vi "16DUT VSA Plot Ver1.0.vi"(6 "Plot":T1(ring), 7 "No of Rows":i32=10496, 8 "error in (no error)":errorcluster, 10 "Bank":enum16{"C1", "C2", "C3"}(ring), 11 "file path (dialog if empty)":path) -> (0 "error out":errorcluster, 3 "Delta C_Min Plot":dbl[][](graph) caption="(Y) Multi Plot 2")   [LabVIEW 2012]
uses:
  <vilib>/Utility/file.llb/Read From Spreadsheet File (string).vi
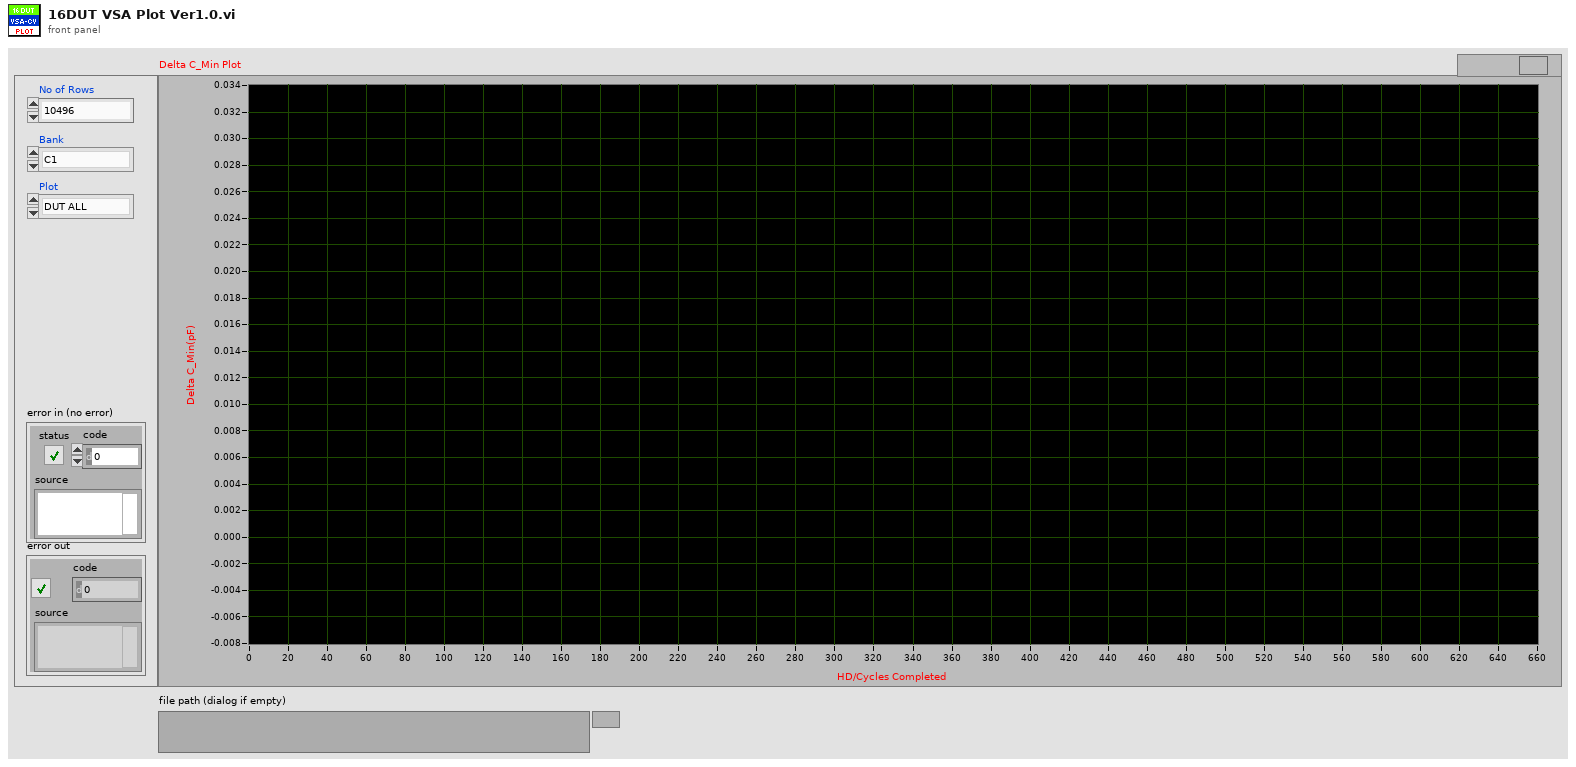
[diagram p1: front panel]
types:
  T1 = enum16{"DUT ALL", "DUT 01", "DUT 02", "DUT 03", "DUT 04", "DUT 05", "DUT 06", "DUT 07", "DUT 08", "DUT 09", "DUT 10", "DUT 11", "DUT 12", "DUT 13", "DUT 14", "DUT 15", "DUT 16"}
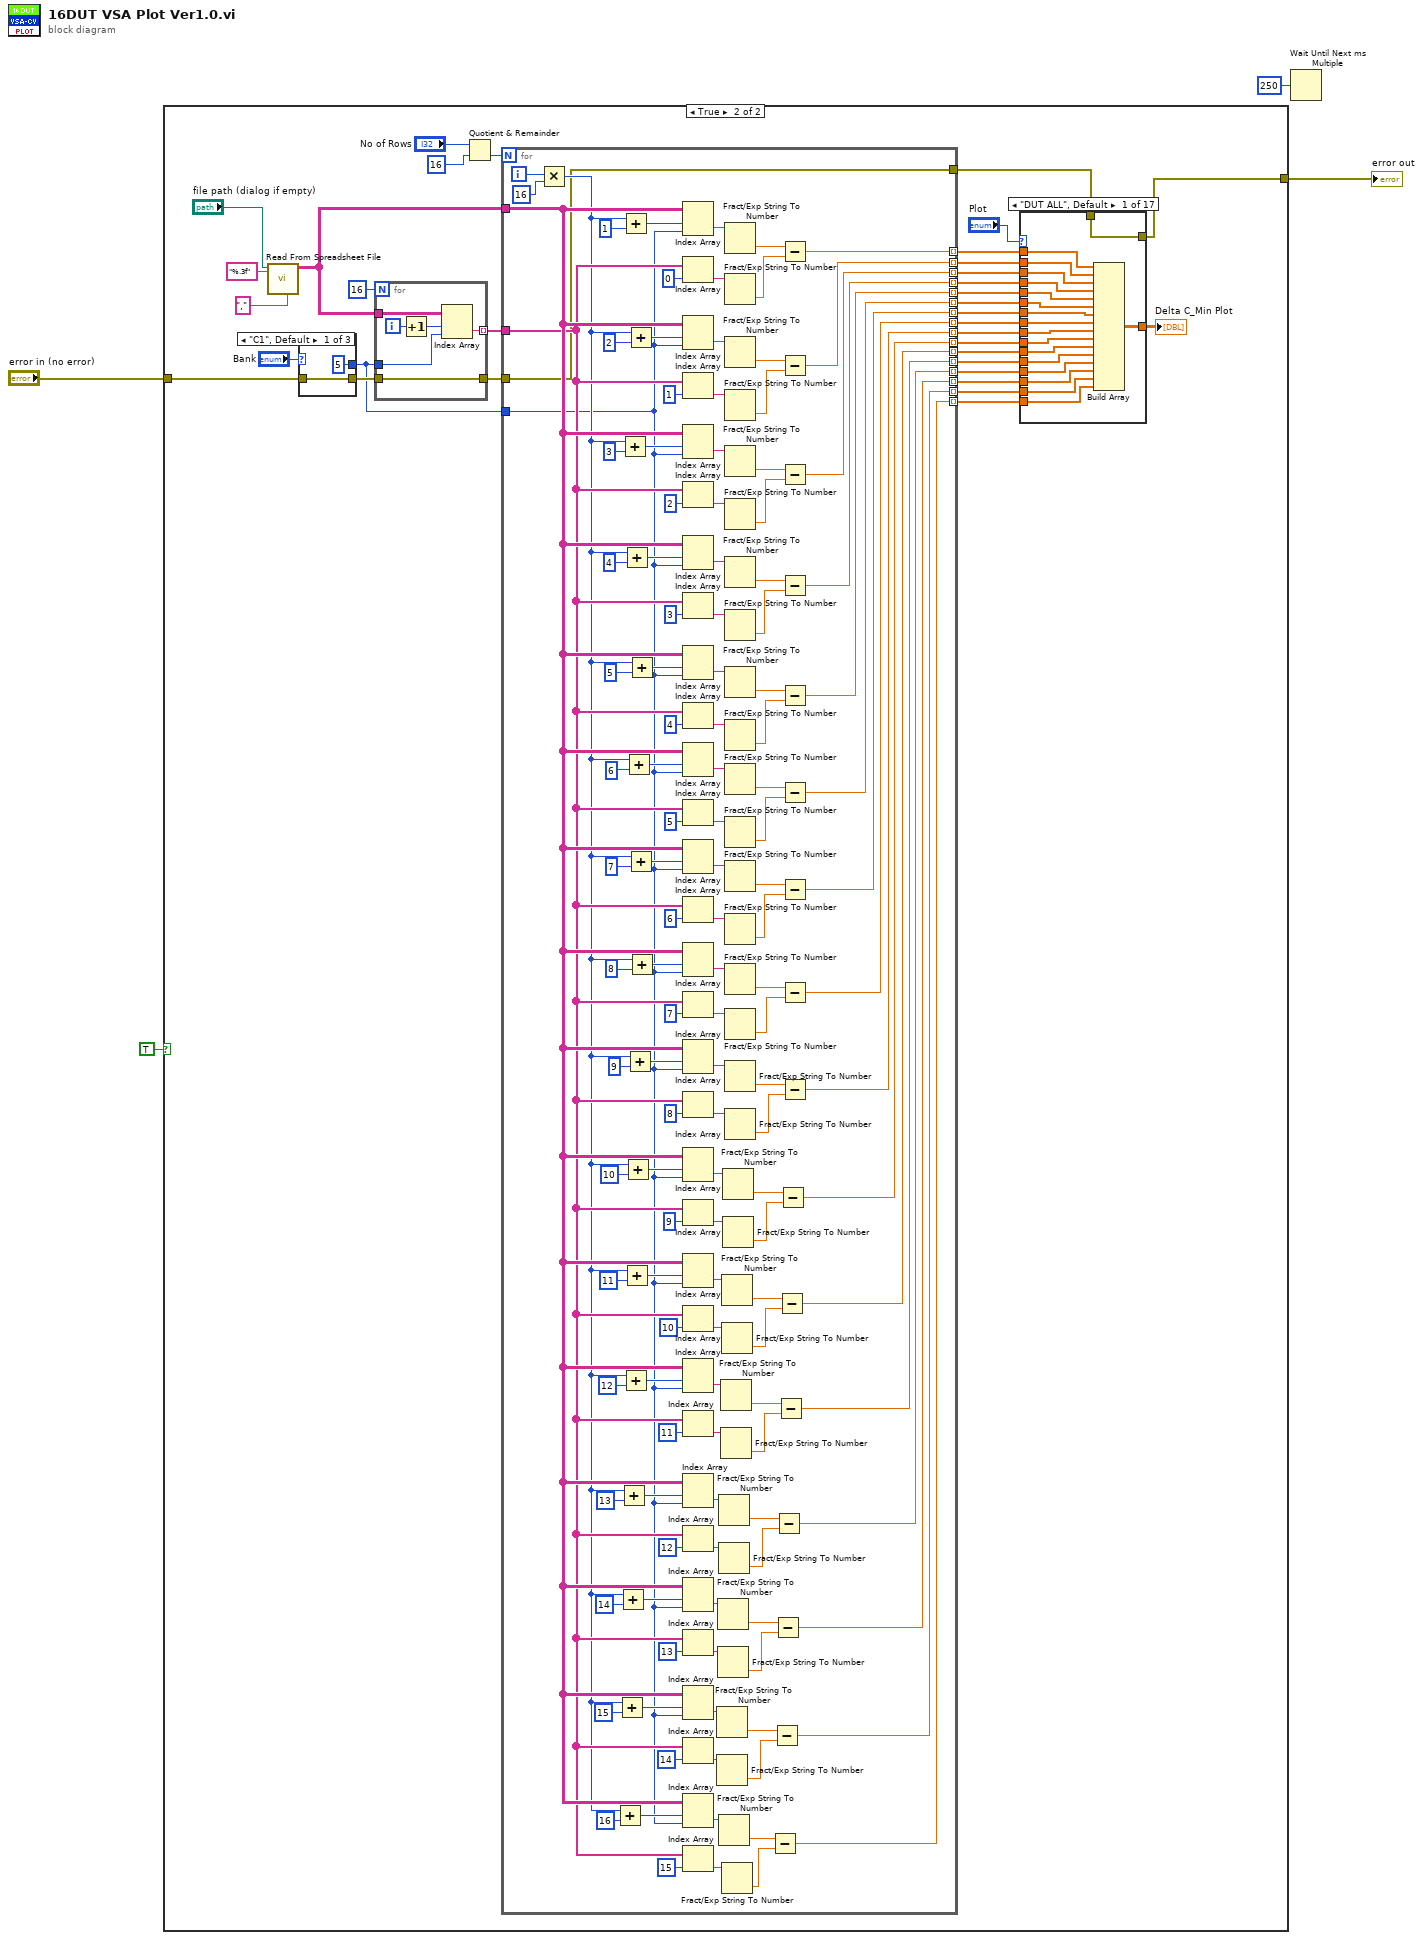
[diagram p0: block diagram]
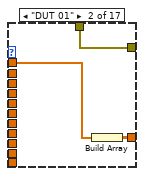
[diagram p3: hidden frame]
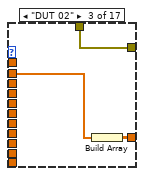
[diagram p4: hidden frame]
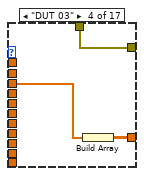
[diagram p5: hidden frame]
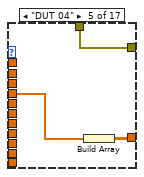
[diagram p6: hidden frame]
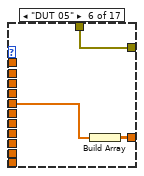
[diagram p7: hidden frame]
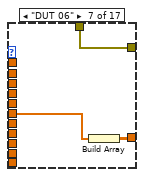
[diagram p8: hidden frame]
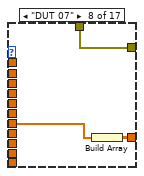
[diagram p9: hidden frame]
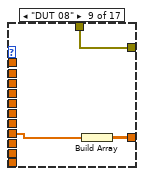
[diagram p10: hidden frame]
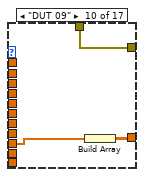
[diagram p11: hidden frame]
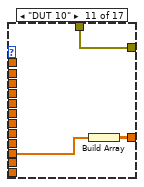
[diagram p12: hidden frame]
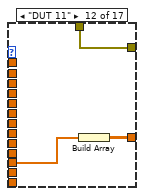
[diagram p13: hidden frame]
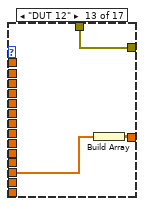
[diagram p14: hidden frame]
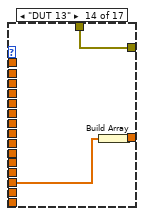
[diagram p15: hidden frame]
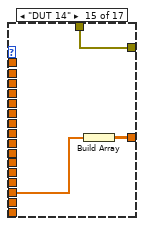
[diagram p16: hidden frame]
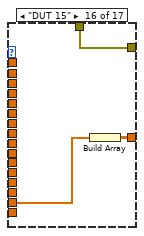
[diagram p17: hidden frame]
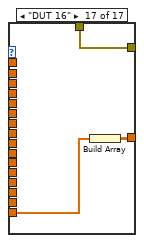
[diagram p18: hidden frame]
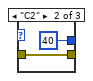
[diagram p19: hidden frame]
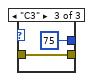
[diagram p20: hidden frame]
diagram:
  n1 = case shown="True" TRUE {
    tunnel: "error in (no error)" -> [w5 w12]
    tunnel: [w5 w6] -> w3
    frame False {
    }
    frame True {
      n2 = call-poly <vilib>:"Read From Spreadsheet File.vi"("delimiter (\\t)"="," ("delimiter (\\t)"), "format (%s)"="%.3f" ("format (%.3f)"), "file path (dialog if empty)"="file path (dialog if empty)") -> ("all rows"=w36:string[][])  [unwired: 4 in, 4 out]
      n3 = case shown="\"C1\", Default" "Bank" {
        tunnel: [5 40 75] -> w8
        tunnel: [w106 w108 w110] -> w9
        tunnel: w12 -> [w106 w108 w110]
        frame "C1", Default {
        }
        frame "C2" {
        }
        frame "C3" {
        }
      }
      n4 = for {
        N: 16 -> [_]
        tunnel: w36 -> [w252]
        tunnel: [w251] -> w35 mode=indexing
        tunnel: w8 -> [w247]
        tunnel: [w248] -> w11
        tunnel: w9 -> [w248]
        i -> [w250]
        n5 = Increment(x=w250) -> (x+1=w249:i32)
        n6 = Index Array(array=w252, index (row)=w249, index (col)=w247) -> (element=w251:string)
      }
      n7 = Quotient & Remainder(x="No of Rows", y=16) -> (floor(x/y)=w31:i32)  [unwired: 1 out]
      n8 = for {
        N: w31 -> [_]
        tunnel: w36 -> [w133]
        tunnel: w35 -> [w132]
        tunnel: [w130] -> w29 mode=indexing
        tunnel: [w129] -> w28 mode=indexing
        tunnel: [w128] -> w27 mode=indexing
        tunnel: [w127] -> w26 mode=indexing
        tunnel: [w126] -> w25 mode=indexing
        tunnel: [w125] -> w24 mode=indexing
        tunnel: [w124] -> w23 mode=indexing
        tunnel: [w123] -> w22 mode=indexing
        tunnel: [w122] -> w21 mode=indexing
        tunnel: [w121] -> w20 mode=indexing
        tunnel: [w120] -> w19 mode=indexing
        tunnel: [w119] -> w18 mode=indexing
        tunnel: [w118] -> w17 mode=indexing
        tunnel: [w117] -> w16 mode=indexing
        tunnel: [w116] -> w15 mode=indexing
        tunnel: [w115] -> w14 mode=indexing
        tunnel: w11 -> [w114]
        tunnel: [w114] -> w10
        tunnel: w8 -> [w113]
        i -> [w112]
        n9 = Multiply(x=w112, y=16) -> (x*y=w131:i32)
        n10 = Add(x=w131, y=16) -> (x+y=w138:i32)
        n11 = Add(x=w131, y=15) -> (x+y=w143:i32)
        n12 = Add(x=w131, y=14) -> (x+y=w152:i32)
        n13 = Add(x=w131, y=13) -> (x+y=w157:i32)
        n14 = Add(x=w131, y=3) -> (x+y=w212:i32)
        n15 = Add(x=w131, y=1) -> (x+y=w234:i32)
        n16 = Add(x=w131, y=12) -> (x+y=w166:i32)
        n17 = Add(x=w131, y=4) -> (x+y=w211:i32)
        n18 = Add(x=w131, y=11) -> (x+y=w171:i32)
        n19 = Add(x=w131, y=10) -> (x+y=w180:i32)
        n20 = Add(x=w131, y=6) -> (x+y=w197:i32)
        n21 = Add(x=w131, y=9) -> (x+y=w227:i32)
        n22 = Add(x=w131, y=2) -> (x+y=w231:i32)
        n23 = Add(x=w131, y=7) -> (x+y=w190:i32)
        n24 = Add(x=w131, y=5) -> (x+y=w204:i32)
        n25 = Add(x=w131, y=8) -> (x+y=w184:i32)
        n26 = Index Array(array=w133, index (row)=w234, index (col)=w113) -> (element=w245:string)
        n27 = Index Array(array=w132, index=0) -> (element=w243:string)
        n28 = Index Array(array=w133, index (row)=w231, index (col)=w113) -> (element=w236:string)
        n29 = Index Array(array=w132, index=1) -> (element=w238:string)
        n30 = Index Array(array=w133, index (row)=w212, index (col)=w113) -> (element=w224:string)
        n31 = Index Array(array=w132, index=2) -> (element=w222:string)
        n32 = Index Array(array=w133, index (row)=w211, index (col)=w113) -> (element=w214:string)
        n33 = Index Array(array=w132, index=3) -> (element=w216:string)
        n34 = Index Array(array=w133, index (row)=w204, index (col)=w113) -> (element=w210:string)
        n35 = Index Array(array=w132, index=4) -> (element=w208:string)
        n36 = Index Array(array=w133, index (row)=w197, index (col)=w113) -> (element=w199:string)
        n37 = Index Array(array=w132, index=5) -> (element=w201:string)
        n38 = Index Array(array=w133, index (row)=w190, index (col)=w113) -> (element=w196:string)
        n39 = Index Array(array=w132, index=6) -> (element=w194:string)
        n40 = Index Array(array=w133, index (row)=w184, index (col)=w113) -> (element=w183:string)
        n41 = Index Array(array=w132, index=7) -> (element=w187:string)
        n42 = Index Array(array=w133, index (row)=w227, index (col)=w113) -> (element=w230:string)
        n43 = Index Array(array=w132, index=8) -> (element=w228:string)
        n44 = Index Array(array=w133, index (row)=w180, index (col)=w113) -> (element=w177:string)
        n45 = Index Array(array=w132, index=9) -> (element=w179:string)
        n46 = Index Array(array=w133, index (row)=w171, index (col)=w113) -> (element=w174:string)
        n47 = Index Array(array=w132, index=10) -> (element=w172:string)
        n48 = Index Array(array=w133, index (row)=w166, index (col)=w113) -> (element=w163:string)
        n49 = Index Array(array=w132, index=11) -> (element=w165:string)
        n50 = Index Array(array=w133, index (row)=w157, index (col)=w113) -> (element=w160:string)
        n51 = Index Array(array=w132, index=12) -> (element=w158:string)
        n52 = Index Array(array=w133, index (row)=w152, index (col)=w113) -> (element=w149:string)
        n53 = Index Array(array=w132, index=13) -> (element=w151:string)
        n54 = Index Array(array=w133, index (row)=w143, index (col)=w113) -> (element=w146:string)
        n55 = Index Array(array=w132, index=14) -> (element=w144:string)
        n56 = Index Array(array=w133, index (row)=w138, index (col)=w113) -> (element=w135:string)
        n57 = Index Array(array=w132, index=15) -> (element=w137:string)
        n58 = Fract/Exp String To Number(string=w146) -> (number=w142:dbl)  [unwired: 3 in, 1 out]
        n59 = Fract/Exp String To Number(string=w144) -> (number=w141:dbl)  [unwired: 3 in, 1 out]
        n60 = Fract/Exp String To Number(string=w149) -> (number=w153:dbl)  [unwired: 3 in, 1 out]
        n61 = Fract/Exp String To Number(string=w151) -> (number=w154:dbl)  [unwired: 3 in, 1 out]
        n62 = Fract/Exp String To Number(string=w160) -> (number=w156:dbl)  [unwired: 3 in, 1 out]
        n63 = Fract/Exp String To Number(string=w158) -> (number=w155:dbl)  [unwired: 3 in, 1 out]
        n64 = Fract/Exp String To Number(string=w135) -> (number=w139:dbl)  [unwired: 3 in, 1 out]
        n65 = Fract/Exp String To Number(string=w163) -> (number=w167:dbl)  [unwired: 3 in, 1 out]
        n66 = Fract/Exp String To Number(string=w165) -> (number=w168:dbl)  [unwired: 3 in, 1 out]
        n67 = Fract/Exp String To Number(string=w174) -> (number=w170:dbl)  [unwired: 3 in, 1 out]
        n68 = Fract/Exp String To Number(string=w172) -> (number=w169:dbl)  [unwired: 3 in, 1 out]
        n69 = Fract/Exp String To Number(string=w137) -> (number=w140:dbl)  [unwired: 3 in, 1 out]
        n70 = Fract/Exp String To Number(string=w177) -> (number=w181:dbl)  [unwired: 3 in, 1 out]
        n71 = Fract/Exp String To Number(string=w179) -> (number=w182:dbl)  [unwired: 3 in, 1 out]
        n72 = Fract/Exp String To Number(string=w245) -> (number=w242:dbl)  [unwired: 3 in, 1 out]
        n73 = Fract/Exp String To Number(string=w243) -> (number=w241:dbl)  [unwired: 3 in, 1 out]
        n74 = Fract/Exp String To Number(string=w236) -> (number=w239:dbl)  [unwired: 3 in, 1 out]
        n75 = Fract/Exp String To Number(string=w238) -> (number=w240:dbl)  [unwired: 3 in, 1 out]
        n76 = Fract/Exp String To Number(string=w224) -> (number=w221:dbl)  [unwired: 3 in, 1 out]
        n77 = Fract/Exp String To Number(string=w222) -> (number=w220:dbl)  [unwired: 3 in, 1 out]
        n78 = Fract/Exp String To Number(string=w214) -> (number=w217:dbl)  [unwired: 3 in, 1 out]
        n79 = Fract/Exp String To Number(string=w216) -> (number=w218:dbl)  [unwired: 3 in, 1 out]
        n80 = Fract/Exp String To Number(string=w210) -> (number=w207:dbl)  [unwired: 3 in, 1 out]
        n81 = Fract/Exp String To Number(string=w208) -> (number=w206:dbl)  [unwired: 3 in, 1 out]
        n82 = Fract/Exp String To Number(string=w199) -> (number=w202:dbl)  [unwired: 3 in, 1 out]
        n83 = Fract/Exp String To Number(string=w201) -> (number=w203:dbl)  [unwired: 3 in, 1 out]
        n84 = Fract/Exp String To Number(string=w196) -> (number=w193:dbl)  [unwired: 3 in, 1 out]
        n85 = Fract/Exp String To Number(string=w194) -> (number=w192:dbl)  [unwired: 3 in, 1 out]
        n86 = Fract/Exp String To Number(string=w183) -> (number=w188:dbl)  [unwired: 3 in, 1 out]
        n87 = Fract/Exp String To Number(string=w187) -> (number=w189:dbl)  [unwired: 3 in, 1 out]
        n88 = Fract/Exp String To Number(string=w230) -> (number=w226:dbl)  [unwired: 3 in, 1 out]
        n89 = Fract/Exp String To Number(string=w228) -> (number=w225:dbl)  [unwired: 3 in, 1 out]
        n90 = Subtract(x=w139, y=w140) -> (x-y=w115:dbl)
        n91 = Subtract(x=w142, y=w141) -> (x-y=w116:dbl)
        n92 = Subtract(x=w153, y=w154) -> (x-y=w117:dbl)
        n93 = Subtract(x=w156, y=w155) -> (x-y=w118:dbl)
        n94 = Subtract(x=w167, y=w168) -> (x-y=w119:dbl)
        n95 = Subtract(x=w170, y=w169) -> (x-y=w120:dbl)
        n96 = Subtract(x=w181, y=w182) -> (x-y=w121:dbl)
        n97 = Subtract(x=w242, y=w241) -> (x-y=w130:dbl)
        n98 = Subtract(x=w239, y=w240) -> (x-y=w129:dbl)
        n99 = Subtract(x=w221, y=w220) -> (x-y=w128:dbl)
        n100 = Subtract(x=w217, y=w218) -> (x-y=w127:dbl)
        n101 = Subtract(x=w207, y=w206) -> (x-y=w126:dbl)
        n102 = Subtract(x=w202, y=w203) -> (x-y=w125:dbl)
        n103 = Subtract(x=w193, y=w192) -> (x-y=w124:dbl)
        n104 = Subtract(x=w188, y=w189) -> (x-y=w123:dbl)
        n105 = Subtract(x=w226, y=w225) -> (x-y=w122:dbl)
      }
      n106 = case shown="\"DUT ALL\", Default" "Plot" {
        tunnel: w29 -> [w57 w60 _ _ _ _ _ _ _ _ _ _ _ _ _ _ _]
        tunnel: w28 -> [w56 _ w62 _ _ _ _ _ _ _ _ _ _ _ _ _ _]
        tunnel: w27 -> [w55 _ _ w66 _ _ _ _ _ _ _ _ _ _ _ _ _]
        tunnel: w26 -> [w54 _ _ _ w68 _ _ _ _ _ _ _ _ _ _ _ _]
        tunnel: w25 -> [w53 _ _ _ _ w72 _ _ _ _ _ _ _ _ _ _ _]
        tunnel: w24 -> [w52 _ _ _ _ _ w74 _ _ _ _ _ _ _ _ _ _]
        tunnel: w23 -> [w51 _ _ _ _ _ _ w77 _ _ _ _ _ _ _ _ _]
        tunnel: w22 -> [w50 _ _ _ _ _ _ _ w81 _ _ _ _ _ _ _ _]
        tunnel: w21 -> [w49 _ _ _ _ _ _ _ _ w84 _ _ _ _ _ _ _]
        tunnel: w20 -> [w48 _ _ _ _ _ _ _ _ _ w87 _ _ _ _ _ _]
        tunnel: w19 -> [w47 _ _ _ _ _ _ _ _ _ _ w90 _ _ _ _ _]
        tunnel: w18 -> [w46 _ _ _ _ _ _ _ _ _ _ _ w93 _ _ _ _]
        tunnel: w17 -> [w45 _ _ _ _ _ _ _ _ _ _ _ _ w96 _ _ _]
        tunnel: w16 -> [w44 _ _ _ _ _ _ _ _ _ _ _ _ _ w99 _ _]
        tunnel: w15 -> [w43 _ _ _ _ _ _ _ _ _ _ _ _ _ _ w102 _]
        tunnel: w14 -> [w42 _ _ _ _ _ _ _ _ _ _ _ _ _ _ _ w104]
        tunnel: [w41 w59 w63 w65 w69 w71 w75 w78 w80 w83 w86 w89 w92 w95 w98 w101 w105] -> w13
        tunnel: w10 -> [w40 w58 w61 w64 w67 w70 w73 w76 w79 w82 w85 w88 w91 w94 w97 w100 w103]
        tunnel: [w40 w58 w61 w64 w67 w70 w73 w76 w79 w82 w85 w88 w91 w94 w97 w100 w103] -> w6
        frame "DUT ALL", Default {
          n107 = Build Array(w57, w56, w55, w54, w53, w52, w51, w50, w49, w48, w47, w46, w45, w44, w43, w42) -> (w41:dbl[][])
        }
        frame "DUT 01" {
          n108 = Build Array(w60) -> (w59:dbl[][])
        }
        frame "DUT 02" {
          n109 = Build Array(w62) -> (w63:dbl[][])
        }
        frame "DUT 03" {
          n110 = Build Array(w66) -> (w65:dbl[][])
        }
        frame "DUT 04" {
          n111 = Build Array(w68) -> (w69:dbl[][])
        }
        frame "DUT 05" {
          n112 = Build Array(w72) -> (w71:dbl[][])
        }
        frame "DUT 06" {
          n113 = Build Array(w74) -> (w75:dbl[][])
        }
        frame "DUT 07" {
          n114 = Build Array(w77) -> (w78:dbl[][])
        }
        frame "DUT 08" {
          n115 = Build Array(w81) -> (w80:dbl[][])
        }
        frame "DUT 09" {
          n116 = Build Array(w84) -> (w83:dbl[][])
        }
        frame "DUT 10" {
          n117 = Build Array(w87) -> (w86:dbl[][])
        }
        frame "DUT 11" {
          n118 = Build Array(w90) -> (w89:dbl[][])
        }
        frame "DUT 12" {
          n119 = Build Array(w93) -> (w92:dbl[][])
        }
        frame "DUT 13" {
          n120 = Build Array(w96) -> (w95:dbl[][])
        }
        frame "DUT 14" {
          n121 = Build Array(w99) -> (w98:dbl[][])
        }
        frame "DUT 15" {
          n122 = Build Array(w102) -> (w101:dbl[][])
        }
        frame "DUT 16" {
          n123 = Build Array(w104) -> (w105:dbl[][])
        }
      }
      "Delta C_Min Plot" <- w13
    }
  }
  "error out" <- w3
  n124 = Wait Until Next ms Multiple(millisecond multiple=u32 250) -> ()  [unwired: 1 out]
